vi "Start Up Options.vi"(7 "No PW Needed (F)":bool) -> (3 "All On":bool)   [LabVIEW 2018]
uses:
  Type/_RT Command.ctl
  Type/_RT Startup Options.ctl
  RT 9607/_RT Global.vi
panel:
  in  "Source Exhaust Low":bool=TRUE
  in  "Out of Gas Flag":bool=TRUE
  in  "System Polling":bool=TRUE
  in  "Turbo Speed":bool=TRUE
  in  "Foreline Pressure":bool=TRUE
  in  "Drying Gas":bool=TRUE
  in  "Door Interlock":bool=TRUE
  in  "Done":bool
  # "For turning on and off the interloack checking sequence during start up."
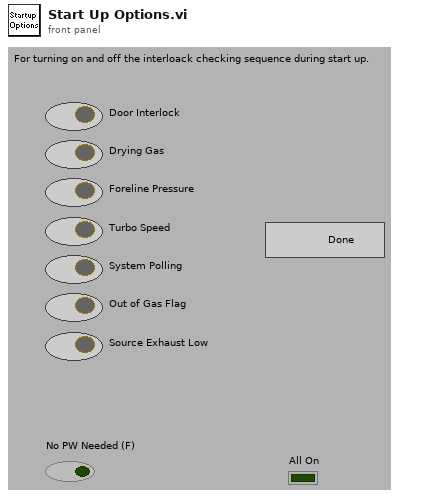
[diagram p1: front panel]
types:
  T1 = typedef "_RT Command.ctl" = enum16{"xml Start Run", "xml Start Actual Run", "xml Stop Run", "xml Runtime Update", "xml Get Status", "xml Get Table", "xml Set Table", "xml Get Configuration", "xml System Status", "xml Set LC Input Logic", "xml Get Data", "xml Get Info", "Start", "StartActualRun", "Stop", "Runtime Update", "Get Data", "Get Info", "Get Status", "Get Param", "Get Config", "Get Table", "Read ADC", "Set Oscillator", "Update Config", "Update Table", "Set All Pol", "Set Pol and DC", "Set Max Mass", "Toggle RP", "Toggle EL", "Set PIC", "Initialize Turbo", "Send Turbo Comm", "Close Turbo", "P1", "P2", "P3", "Send Serial", "Set LC Out", "Get LC In", "Read VAC", "Test Table", "Toggle Power", "Get Startup", "Set Startup", "Get ADC Table", "Set ADC Table", "Get Brief Status", "Get Detail Status", "Auxiliary Update", "Set CC Logics", "Set CC Input Logics", "Ignore Error", "invalid"}
  T2 = typedef "_RT Startup Options.ctl" = cluster{"Door":bool, "Curtain":bool, "Pressure":bool, "Turbo":bool, "SysPoll":bool, "GasFlag":bool, "SourceExhaust":bool}
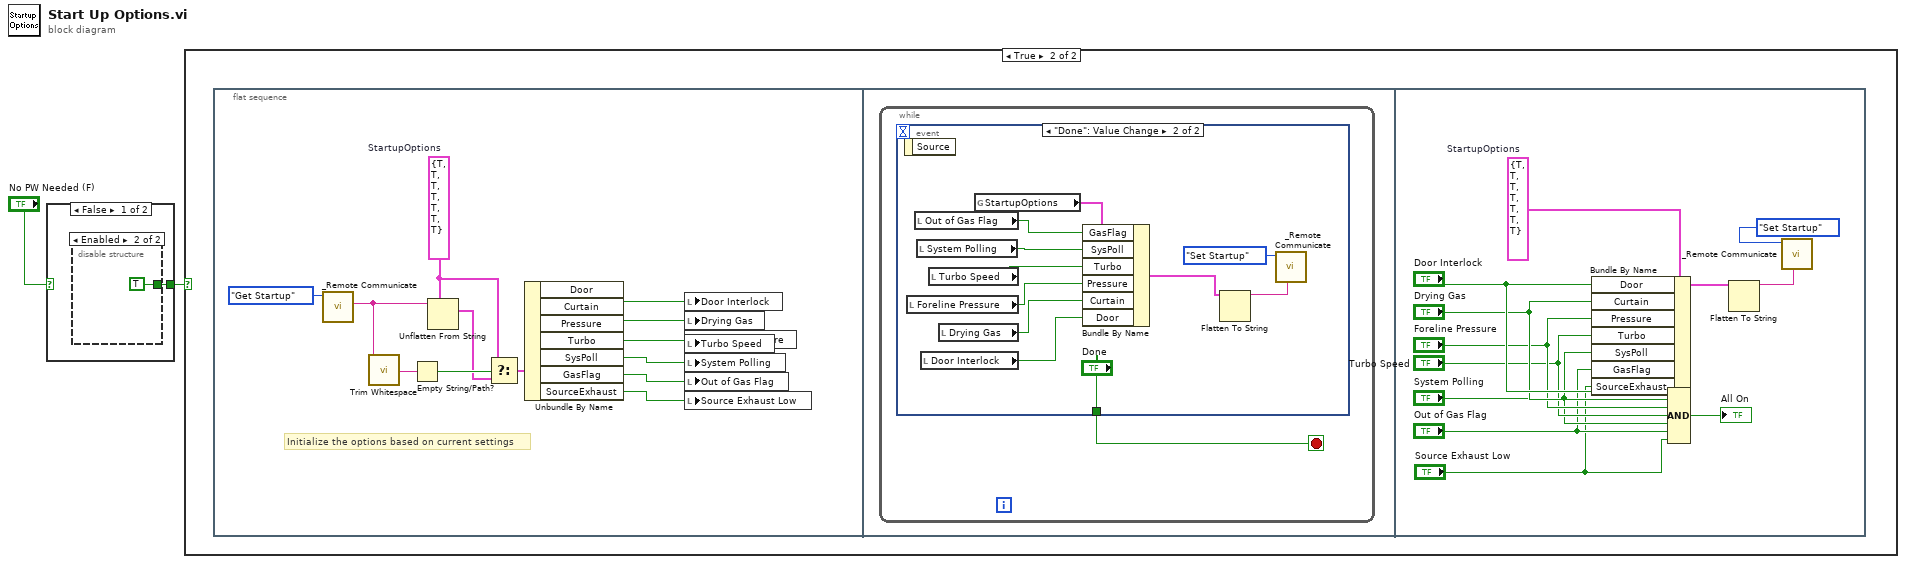
[diagram p0: block diagram]
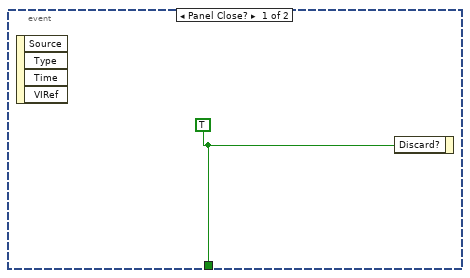
[diagram p3: hidden frame]
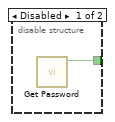
[diagram p4: hidden frame]
diagram:
  n1 = case shown="False" "No PW Needed (F)" {
    selector: "No PW Needed (F)" -> [_ w6]
    tunnel: [w3 w6] -> w2
    frame False {
      n2 = disable-structure shown="Enabled" {
        disable-tunnel: [w4 TRUE ("Valid")] -> w3
        frame Disabled {
          n3 = call "Get Password.vi"() -> ("Valid"=w4:bool)  [unwired: 1 in, 6 out]
        }
        frame Enabled {
        }
      }
    }
    frame True {
    }
  }
  n4 = case shown="True" w2 {
    frame False {
    }
    frame True {
      n5 = flat-sequence {
        frame #0 {
          w13 = T2 {"Door"=TRUE, "Curtain"=TRUE, "Pressure"=TRUE, "Turbo"=TRUE, "SysPoll"=TRUE, "GasFlag"=TRUE, "SourceExhaust"=TRUE}  # StartupOptions
          # "Initialize the options based on current settings"
          n6 = call "_Remote Communicate.vi"("Command"=_RT_Command."Get Startup") -> ("Info"=w16:string)  [unwired: 5 in, 3 out]
          n7 = call <vilib>:"Trim Whitespace.vi"("string"=w16) -> ("trimmed string"=w15:string)  [unwired: 1 in]
          n8 = Empty String/Path?(string/path=w15) -> (empty?=w14:bool)
          n9 = Unflatten From String(type=w13, binary string=w16) -> (value=w12:T2)  [unwired: 1 in, 4 out]
          n10 = Select(t=w13, s=w14, f=w12) -> (s? t:f=w11:T2)
          n11 = Unbundle By Name(w11) -> ("Door"=w19:bool, "Curtain"=w18:bool, "Pressure"=w10:bool, "Turbo"=w17:bool, "SysPoll"=w9:bool, "GasFlag"=w8:bool, "SourceExhaust"=w7:bool)
          n12 = local write "Door Interlock"(w19) -> ()
          n13 = local write "Drying Gas"(w18) -> ()
          n14 = local write "Foreline Pressure"(w10) -> ()
          n15 = local write "Turbo Speed"(w17) -> ()
          n16 = local write "System Polling"(w9) -> ()
          n17 = local write "Out of Gas Flag"(w8) -> ()
          n18 = local write "Source Exhaust Low"(w7) -> ()
        }
        frame #1 {
          n19 = while {
            stop <- w21 stop-if-true
            n20 = event shown="[1] \"Done\": Value Change" {
              selector: _ -> [_ _]
              dyn-events: _ -> [_ _]
              timeout: _ -> [_ _]
              tunnel: [w22 "Done"] -> w21
              event Panel Close? {
                w22 = TRUE
                n21 = event-data() -> ()  [unwired: 5 out]
                n22 = event-data("Discard?"=w22) -> ()  [unwired: 1 in, 1 out]
              }
              event "Done": Value Change {
                n23 = event-data() -> ()  [unwired: 2 out]
                n24 = local read "Foreline Pressure"() -> (w30:bool)
                n25 = local read "Out of Gas Flag"() -> (w27:bool)
                n26 = local read "System Polling"() -> (w28:bool)
                n27 = local read "Door Interlock"() -> (w23:bool)
                n28 = local read "Turbo Speed"() -> (w29:bool)
                n29 = local read "Drying Gas"() -> (w31:bool)
                n30 = global read "_RT Global.vi" "StartupOptions"() -> (w24:T2)
                n31 = Bundle By Name(cluster=w24, "GasFlag"=w27, "SysPoll"=w28, "Turbo"=w29, "Pressure"=w30, "Curtain"=w31, "Door"=w23) -> (w26:T2)
                n32 = Flatten To String(anything=w26) -> (data string=w25:string)  [unwired: 3 in, 2 out]
                n33 = call "_Remote Communicate.vi"("String"=w25, "Command"=_RT_Command."Set Startup") -> ()  [unwired: 4 in, 4 out]
              }
            }
          }
        }
        frame #2 {
          w42 = T2 {"Door"=TRUE, "Curtain"=TRUE, "Pressure"=TRUE, "Turbo"=TRUE, "SysPoll"=TRUE, "GasFlag"=TRUE, "SourceExhaust"=TRUE}  # StartupOptions
          n34 = Bundle By Name(cluster=w42, "Door"="Door Interlock", "Curtain"="Drying Gas", "Pressure"="Foreline Pressure", "Turbo"="Turbo Speed", "SysPoll"="System Polling", "GasFlag"="Out of Gas Flag", "SourceExhaust"="Source Exhaust Low") -> (w45:T2)
          n35 = Compound Arithmetic op=AND("Door Interlock", "Drying Gas", "Foreline Pressure", "Turbo Speed", "System Polling", "Out of Gas Flag", "Source Exhaust Low") -> (→"All On":bool)
          n36 = Flatten To String(anything=w45) -> (data string=w44:string)  [unwired: 1 in, 4 out]
          n37 = call "_Remote Communicate.vi"("String"=w44, "Command"=_RT_Command."Set Startup") -> ()  [unwired: 4 in, 4 out]
        }
      }
    }
  }
